vi "Reattach Notes.vi"(8 "error in (no error)":errorcluster, 11 "sr clusters in":T1[](array[typedef]) {"Creation Date" format="%<%x>T"; "Last Updated" format="%<%x>T"}) -> (0 "error out":errorcluster, 3 "sr clusters out":T1[](array[typedef]) {"Creation Date" format="%<%x>T"; "Last Updated" format="%<%x>T"})   [LabVIEW 2018]
uses:
  Type Defs/SR Cluster.ctl
  Type Defs/SR Status.ctl
  Type Defs/FGV States.ctl
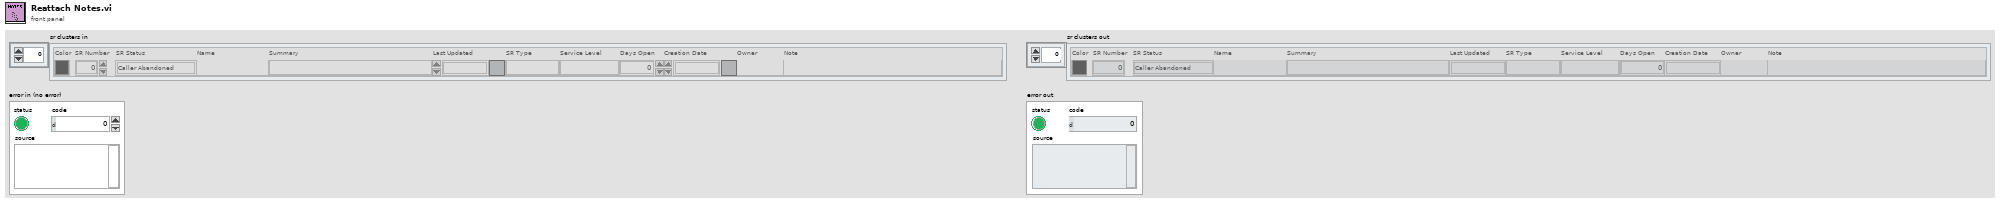
[diagram p1: front panel]
types:
  T1 = typedef "SR Cluster.ctl" = cluster{"Color":u32, "SR Number":i32, "SR Status":T2, "Name":string, "Summary":string, "Last Updated":timestamp, "SR Type":string, "Service Level":string, "Days Open":dbl, "Creation Date":timestamp, "Owner":string, "Note":string}
  T2 = typedef "SR Status.ctl" = enum16{"Caller Abandoned", "Created in Error", "Expired", "Forum Resolved AE", "Forum Resolved Customer", "IN WORK", "IN WORK Collab with AES", "IN WORK Collab with PSE", "IN WORK Collab with SE", "IN WORK Customer Added Note", "IN WORK Escalation", "IN WORK Wait on Customer", "Open", "Potentially Resolved", "Presumed Resolved", "RMA Approved for Return", "RMA Closed", "RMA Closed - DOA", "RMA In Progress", "RMA Open", "RMA Waiting on Customer", "Resolved", "Passed Off"}
  T3 = typedef "FGV States.ctl" = enum16{"Initialize", "Merge", "Write", "Remove", "Read", "Clear"}
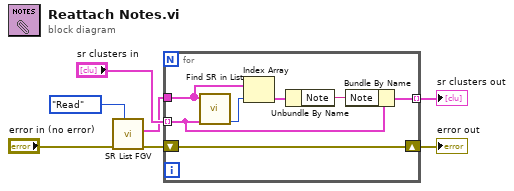
[diagram p0: block diagram]
diagram:
  n1 = call "SR List FGV.vi"("Operation"=FGV_States."Read", "Error In"="error in (no error)") -> ("Error Out"=w2:errorcluster, "list out"=w1:T1[])  [unwired: 8 in]
  n2 = for {
    tunnel: [w8] -> w5 mode=indexing
    tunnel: "sr clusters in" -> [w9] mode=indexing
    shift-right: [w14] -> w7
    shift-left: w2 -> [w14]
    tunnel: w1 -> [w13]
    n3 = call "Find SR in List.vi"("new SR"=w9, "SR list in"=w13) -> ("SR Index"=w12:i32)  [unwired: 8 in, 1 out]
    n4 = Index Array(array=w13, index=w12) -> (element=w11:T1)
    n5 = Unbundle By Name(w11) -> ("Note"=w10:string)
    n6 = Bundle By Name(cluster=w9, "Note"=w10) -> (w8:T1)
  }
  "error out" <- w7
  "sr clusters out" <- w5
